vi "define active channels.vi"() -> (0 "active channels":i16, 1 "total channel count":i32, 3 "Active channels":T1)   [LabVIEW 2018]
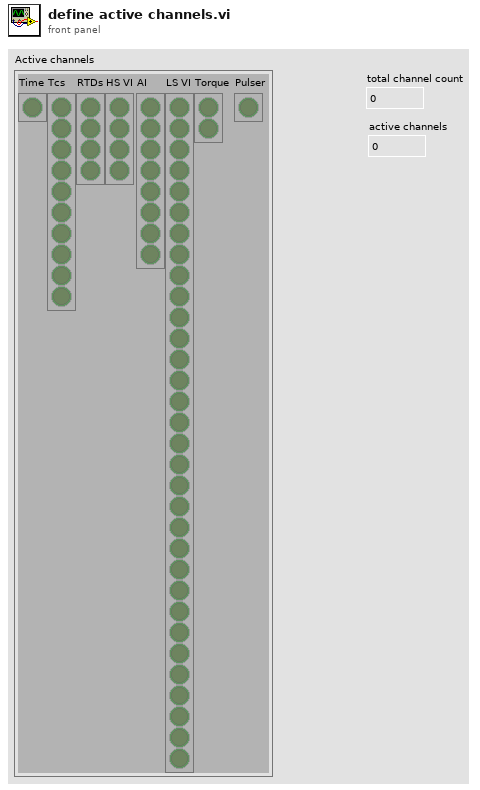
[diagram p1: front panel]
types:
  T1 = cluster{"Time":bool[], "Tcs":bool[], "RTDs":bool[], "HS VI":bool[], "AI":bool[], "LS VI":bool[], "Torque":bool[], "Pulser":bool[]}
  T2 = cluster{"Torque":bool[], "Time":bool[], "Tcs":bool[], "RTDs":bool[], "HS VI":bool[], "AI":bool[], "LS VI":bool[], "Pulser":bool[]}
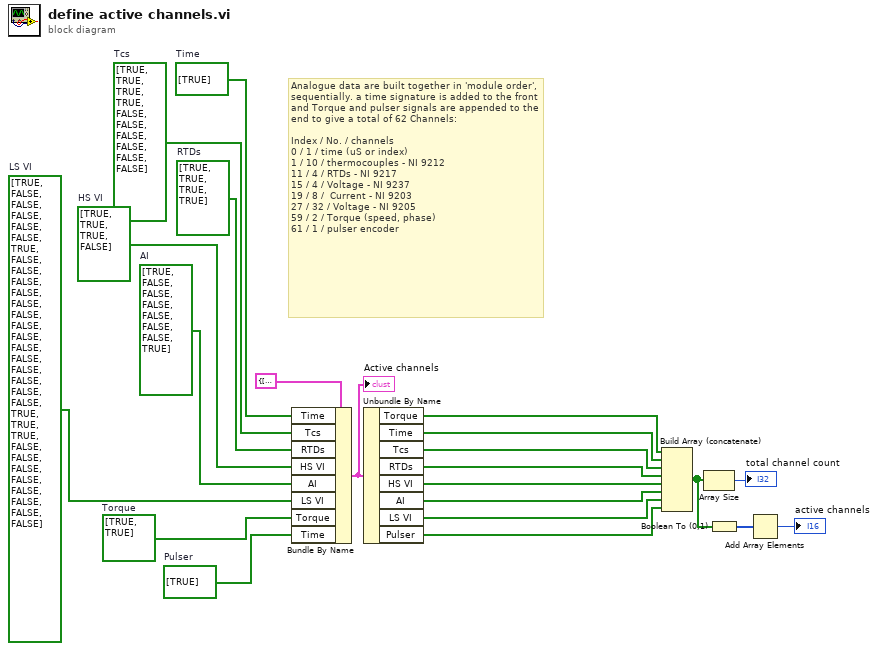
[diagram p0: block diagram]
diagram:
  w4 = bool[] [TRUE]  # Pulser
  w6 = bool[] [TRUE, FALSE, FALSE, FALSE, FALSE, FALSE, TRUE, FALSE, FALSE, FALSE, FALSE, FALSE, FALSE, FALSE, FALSE, FALSE, FALSE, FALSE, FALSE, FALSE, FALSE, TRUE, TRUE, TRUE, FALSE, FALSE, FALSE, FALSE, FALSE, FALSE, FALSE, FALSE]  # LS VI
  w7 = bool[] [TRUE, FALSE, FALSE, FALSE, FALSE, FALSE, FALSE, TRUE]  # AI
  w8 = bool[] [TRUE, TRUE, TRUE, FALSE]  # HS VI
  w9 = bool[] [TRUE, TRUE, TRUE, TRUE]  # RTDs
  w10 = bool[] [TRUE, TRUE, TRUE, TRUE, FALSE, FALSE, FALSE, FALSE, FALSE, FALSE]  # Tcs
  w11 = bool[] [TRUE]  # Time
  w5 = bool[] [TRUE, TRUE]  # Torque
  # "Analogue data are built together in 'module order', sequentially. a time signature is added to the front and Torque and pulser signals are appended to the end to give a total of 62 Channels:\n\nIndex / No. / channels\n0 / 1 / time (uS or index)\n1 / 10 / thermocouples - NI 9212\n11 / 4 / RTDs - NI 9217\n15 / 4 / Voltage - NI 9237\n19 / 8 /  Current - NI 9203\n27 / 32 / Voltage - NI 9205\n59 / 2 / Torque (speed, phase)\n61 / 1 / pulser encoder"
  n1 = Bundle By Name(cluster=T2 {"Torque"=[TRUE, TRUE], "Time"=[TRUE], "Tcs"=[TRUE, TRUE, TRUE, TRUE, FALSE, FALSE, FALSE, FALSE, FALSE, FALSE], "RTDs"=[TRUE, TRUE, TRUE, TRUE], "HS VI"=[TRUE, TRUE, TRUE, FALSE], "AI"=[TRUE, FALSE, FALSE, FALSE, FALSE, FALSE, FALSE, TRUE], "LS VI"=[TRUE, FALSE, FALSE, FALSE, FALSE, FALSE, TRUE, FALSE, FALSE, FALSE, FALSE, FALSE, FALSE, FALSE, FALSE, FALSE, FALSE, FALSE, FALSE, FALSE, FALSE, TRUE, TRUE, TRUE, FALSE, FALSE, FALSE, FALSE, FALSE, FALSE, FALSE, FALSE], "Pulser"=[TRUE]} ("Active channels"), "Time"=w11, "Tcs"=w10, "RTDs"=w9, "HS VI"=w8, "AI"=w7, "LS VI"=w6, "Torque"=w5, "Time"=w4) -> (w12:T2)
  "Active channels" <- w12
  n2 = Unbundle By Name(w12) -> ("Torque"=w21:bool[], "Time"=w20:bool[], "Tcs"=w19:bool[], "RTDs"=w18:bool[], "HS VI"=w17:bool[], "AI"=w16:bool[], "LS VI"=w15:bool[], "Pulser"=w13:bool[])
  n3 = Build Array (concatenate)(w21, w20, w19, w18, w17, w16, w15, w13) -> (w3:bool[])
  n4 = Array Size(array=w3) -> (size(s)=→"total channel count":i32)
  n5 = Boolean To (0,1)(Boolean=w3) -> (0, 1=w2:i16[])
  n6 = Add Array Elements(numeric array=w2) -> (sum=→"active channels":i16)
